vi "TAT_PLC_Data_read.vi"(7 "Enum":enum16{"Read", "Write"}(ring), 8 "error in (no error)":errorcluster, 10 "Array":u16[](array[numeric])) -> (0 "error out":errorcluster, 2 "Array 2":u16[](array[numeric]))   [LabVIEW 2017]
panel:
  # "STATION 1"
  # "SR.NO\tFROM PLC DATA\tDESCRIPTION\tTO SOFTWARE DATA\t\n1\tD604\tCYCLE TIME\tD1030\tD1030\n2\tD1032\tOK COUNTER\tD1032\tD1032\n3\tD1034\tNG COUNTER\tD1043\tD1034\n4"
  # "CONTROL PROCESS TO  LABVIEW from PLC"
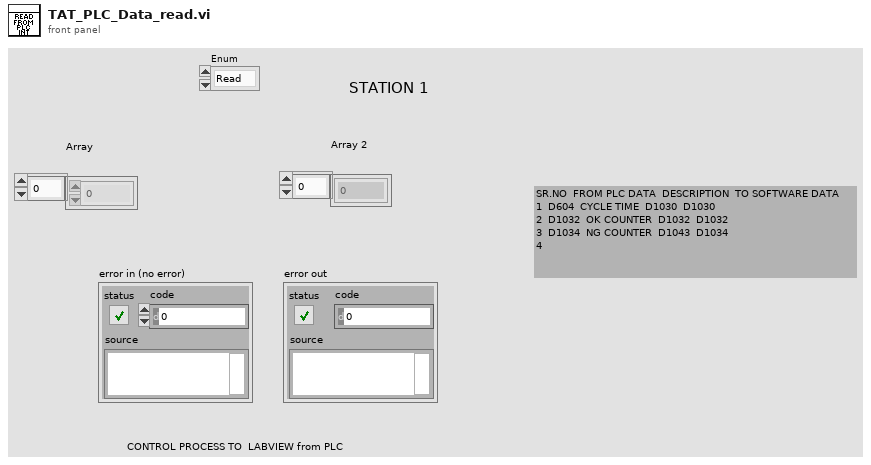
[diagram p1: front panel]
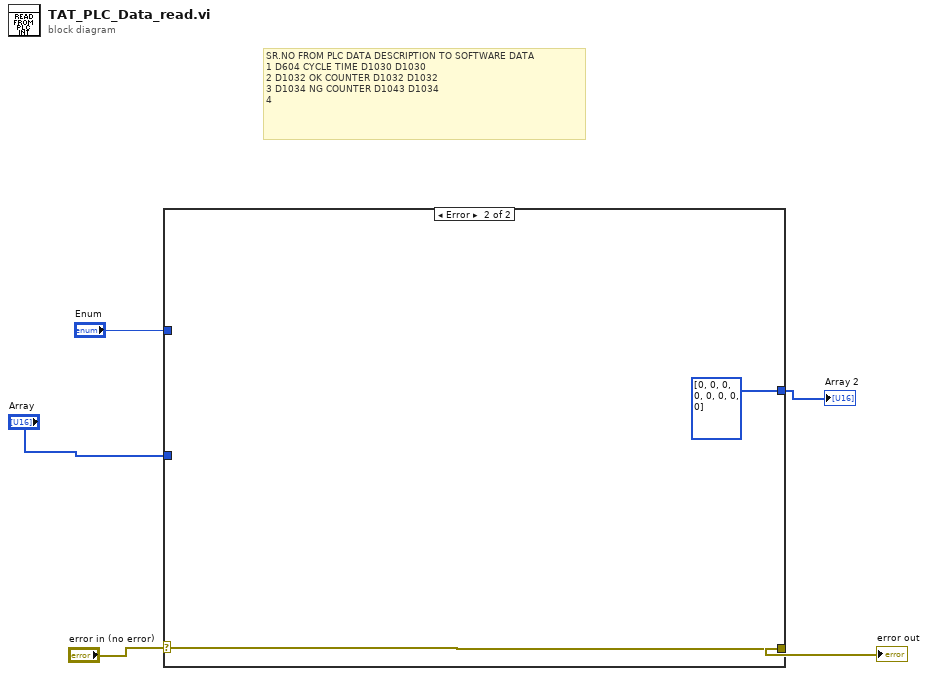
[diagram p0: block diagram]
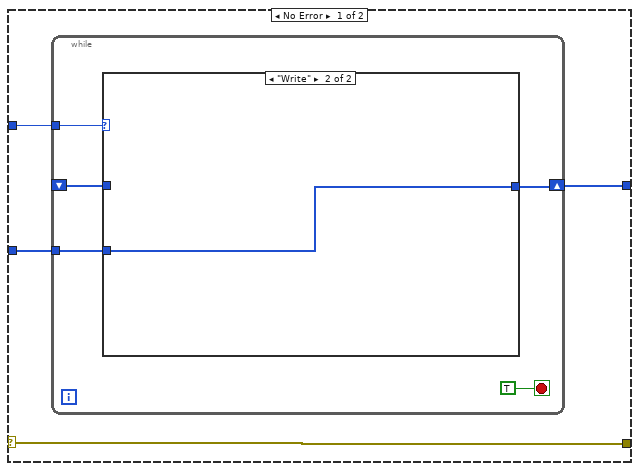
[diagram p2: hidden frame]
diagram:
  # "SR.NO\tFROM PLC DATA\tDESCRIPTION\tTO SOFTWARE DATA\t\n1\tD604\tCYCLE TIME\tD1030\tD1030\n2\tD1032\tOK COUNTER\tD1032\tD1032\n3\tD1034\tNG COUNTER\tD1043\tD1034\n4"
  n1 = case shown="Error" "error in (no error)" {
    selector: "error in (no error)" -> [w6 w18]
    tunnel: [w6 w18] -> w5
    tunnel: "Enum" -> [w9 _]
    tunnel: "Array" -> [w8 _]
    tunnel: [w7 u16[] [0, 0, 0, 0, 0, 0, 0, 0]] -> w1
    frame No Error {
      n2 = while {
        tunnel: w9 -> [w13]
        shift-right: [w10] -> w7
        shift-left: _ -> [w11]
        tunnel: w8 -> [w12]
        stop <- TRUE stop-if-true
        n3 = case shown="\"Write\"" w13 {
          tunnel: w12 -> [_ w16]
          tunnel: [w15 w16] -> w10
          tunnel: w11 -> [w15 _]
          frame "Read", Default {
          }
          frame "Write" {
          }
        }
      }
    }
    frame Error {
    }
  }
  "error out" <- w5
  "Array 2" <- w1
